vi "error_check_shutdown_sweep_field.vi"(8 "State In":T1, 11 "Boolean":bool) -> (3 "State Out":T1)   [LabVIEW 2017]
uses:
  Controls/State.ctl
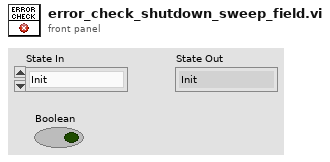
[diagram p1: front panel]
types:
  T1 = typedef "State.ctl" = enum16{"Init", "Idle", "Sweeping up", "Sweeping down", "Running", "Running first time", "Running down", "Shutdown"}
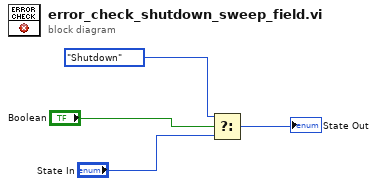
[diagram p0: block diagram]
diagram:
  n1 = Select(t=State."Shutdown", s="Boolean", f="State In") -> (s? t:f=→"State Out":T1)
